vi "Create.vi"(8 "error in (no error)":errorcluster, 11 "QueueMessenger in":refnum<class "QueueMessenger.lvclass">) -> (0 "error out":errorcluster, 3 "QueueMessenger out":refnum<class "QueueMessenger.lvclass">)   [LabVIEW 2011, in "Messenging.lvlib" / "QueueMessenger.lvclass"]
uses:
  QueueMessenger.lvclass
  TextVarientMessage/MSG.lvclass
  QueueMessenger.lvclass/QueueMessenger.ctl
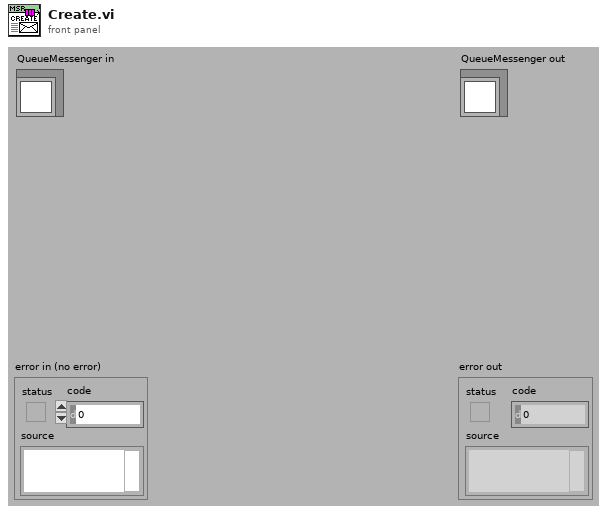
[diagram p1: front panel]
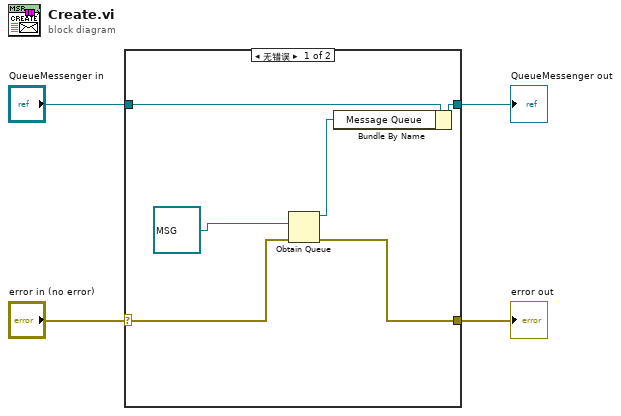
[diagram p0: block diagram]
diagram:
  n1 = case shown="无错误" "error in (no error)" {
    selector: "error in (no error)" -> [w6 w12]
    tunnel: [w5 w12] -> w3
    tunnel: "QueueMessenger in" -> [w10 w11]
    tunnel: [w8 w11] -> w1
    frame No Error {
      n2 = Obtain Queue(element data type=refnum<class "MSG.lvclass"> refnum ("Interprocess Message"), error in (no error)=w6) -> (queue out=w7:refnum<queue>, error out=w5:errorcluster)  [unwired: 2 in, 2 out]
      n3 = Bundle By Name(cluster=w10, "Message Queue"=w7) -> (w8:refnum<class "QueueMessenger.lvclass">)
    }
    frame Error {
    }
  }
  "error out" <- w3
  "QueueMessenger out" <- w1
